vi "ParseHeaderInfo.vi"(2 "Path In":path, 3 "Header Lines":string[](array[string])) -> (1 "Parameters":T1 {"Time" format="%<%H:%M\n%d/%m/%y>T"})   [LabVIEW 2014]
uses:
  <userlib>/CurtinCode/SettingsControl.ctl
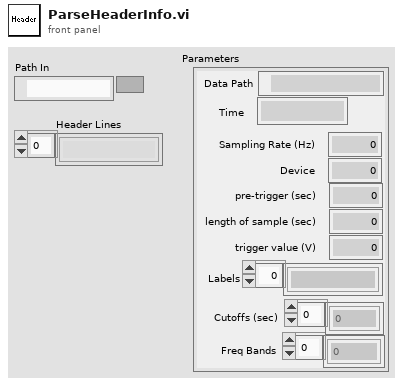
[diagram p1: front panel]
types:
  T1 = typedef "SettingsControl.ctl" = cluster{"Data Path":path, "Time":timestamp, "Sampling Rate (Hz)":u16, "Device":u16, "pre-trigger (sec)":dbl, "length of sample (sec)":dbl, "trigger value (V)":dbl, "Labels":string[], "Cutoffs (sec)":dbl[], "Freq Bands":dbl[]}
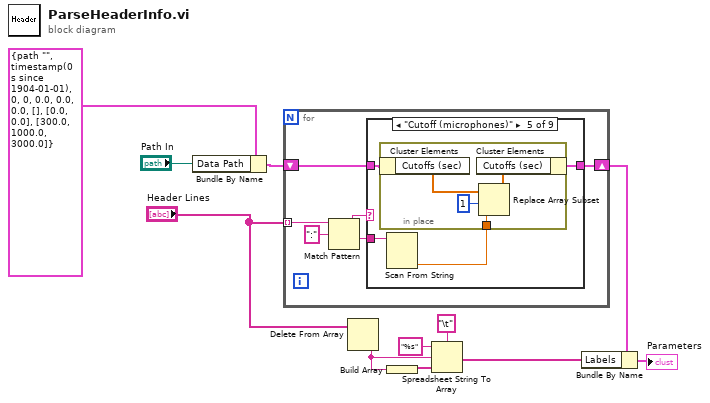
[diagram p0: block diagram]
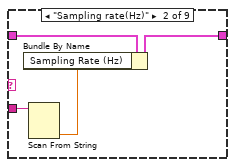
[diagram p3: hidden frame]
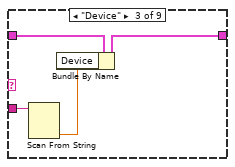
[diagram p4: hidden frame]
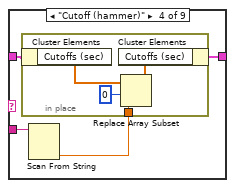
[diagram p5: hidden frame]
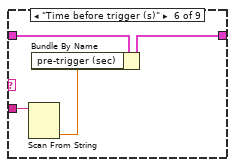
[diagram p6: hidden frame]
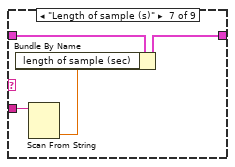
[diagram p7: hidden frame]
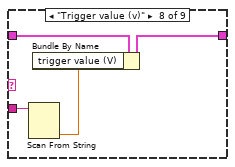
[diagram p8: hidden frame]
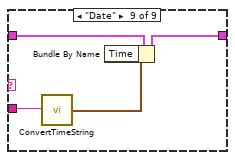
[diagram p9: hidden frame]
diagram:
  n1 = Bundle By Name(cluster=T1 {"Data Path"=path "", "Time"=timestamp(0 s since 1904-01-01), "Sampling Rate (Hz)"=0, "Device"=0, "pre-trigger (sec)"=0.0, "length of sample (sec)"=0.0, "trigger value (V)"=0.0, "Labels"=[], "Cutoffs (sec)"=[0.0, 0.0], "Freq Bands"=[300.0, 1000.0, 3000.0]} ("Parameters"), "Data Path"="Path In") -> (w10:T1)
  n2 = for {
    tunnel: "Header Lines" -> [w17] mode=indexing
    shift-right: [w12] -> w8
    shift-left: w10 -> [w13]
    n3 = Match Pattern(string=w17, regular expression=":") -> (before substring=w15:string, after substring=w14:string)  [unwired: 1 in, 2 out]
    n4 = case shown="\"Cutoff (microphones)\"" w15 {
      tunnel: w14 -> [_ w22 w26 w30 w38 w46 w50 w54 w58]
      tunnel: w13 -> [w18 w21 w25 w29 w37 w45 w49 w53 w57]
      tunnel: [w18 w20 w24 w28 w36 w44 w48 w52 w56] -> w12
      frame Default {
      }
      frame "Sampling rate(Hz)" {
        n5 = Scan From String(input string=w22) -> (output 1=w19:dbl)  [unwired: 4 in, 3 out]
        n6 = Bundle By Name(cluster=w21, "Sampling Rate (Hz)"=w19) -> (w20:T1)
      }
      frame "Device" {
        n7 = Scan From String(input string=w26) -> (output 1=w23:dbl)  [unwired: 4 in, 3 out]
        n8 = Bundle By Name(cluster=w25, "Device"=w23) -> (w24:T1)
      }
      frame "Cutoff (hammer)" {
        n9 = Scan From String(input string=w30) -> (output 1=w27:dbl)  [unwired: 4 in, 3 out]
        n10 = in-place {
          in-place-border: w27 -> [w31]
          n11 = in-place-cluster #1(w29) -> ("Cutoffs (sec)"=w34:dbl[])
          n12 = Replace Array Subset(array=w34, new element=w31, index=0) -> (w33:dbl[])
          n13 = in-place-cluster #1("Cutoffs (sec)"=w33) -> (w28:T1)
        }
      }
      frame "Cutoff (microphones)" {
        n14 = Scan From String(input string=w38) -> (output 1=w35:dbl)  [unwired: 4 in, 3 out]
        n15 = in-place {
          in-place-border: w35 -> [w39]
          n16 = in-place-cluster #2(w37) -> ("Cutoffs (sec)"=w42:dbl[])
          n17 = Replace Array Subset(array=w42, new element=w39, index=1) -> (w41:dbl[])
          n18 = in-place-cluster #2("Cutoffs (sec)"=w41) -> (w36:T1)
        }
      }
      frame "Time before trigger (s)" {
        n19 = Scan From String(input string=w46) -> (output 1=w43:dbl)  [unwired: 4 in, 3 out]
        n20 = Bundle By Name(cluster=w45, "pre-trigger (sec)"=w43) -> (w44:T1)
      }
      frame "Length of sample (s)" {
        n21 = Scan From String(input string=w50) -> (output 1=w47:dbl)  [unwired: 4 in, 3 out]
        n22 = Bundle By Name(cluster=w49, "length of sample (sec)"=w47) -> (w48:T1)
      }
      frame "Trigger value (v)" {
        n23 = Scan From String(input string=w54) -> (output 1=w51:dbl)  [unwired: 4 in, 3 out]
        n24 = Bundle By Name(cluster=w53, "trigger value (V)"=w51) -> (w52:T1)
      }
      frame "Date" {
        n25 = call <userlib>:"ConvertTimeString.vi"("String"=w58) -> ("time stamp"=w55:timestamp)
        n26 = Bundle By Name(cluster=w57, "Time"=w55) -> (w56:T1)
      }
    }
  }
  n27 = Delete From Array(array="Header Lines") -> (deleted portion=w6:string)  [unwired: 2 in, 1 out]
  n28 = Build Array(w6) -> (w7:string[])
  n29 = Spreadsheet String To Array(delimiter (Tab)="\t", format string="%s", spreadsheet string=w6, array type (2D Dbl)=w7) -> (array=w9:string[])
  n30 = Bundle By Name(cluster=w8, "Labels"=w9) -> (→"Parameters":T1)
